vi "split_channels_syncBeforecnt.vi"(7 "last_sync_num_in":i32, 8 "error constant":errorcluster, 9 "sync_channel":u32, 10 "channels":u32[](array[numeric]), 11 "stamps":i64[](array[numeric])) -> (0 "error IO":errorcluster, 1 "time_delays":i64[](array[numeric]), 2 "n_sync":i32[](array[numeric]), 3 "count_channels":u32[](array[numeric]), 5 "last_sync_num_out":i32)   [LabVIEW 2018]
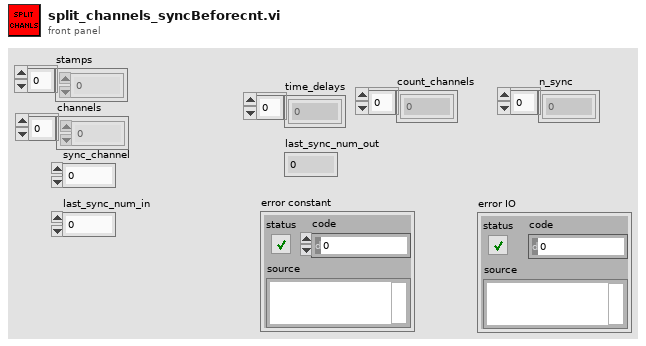
[diagram p1: front panel]
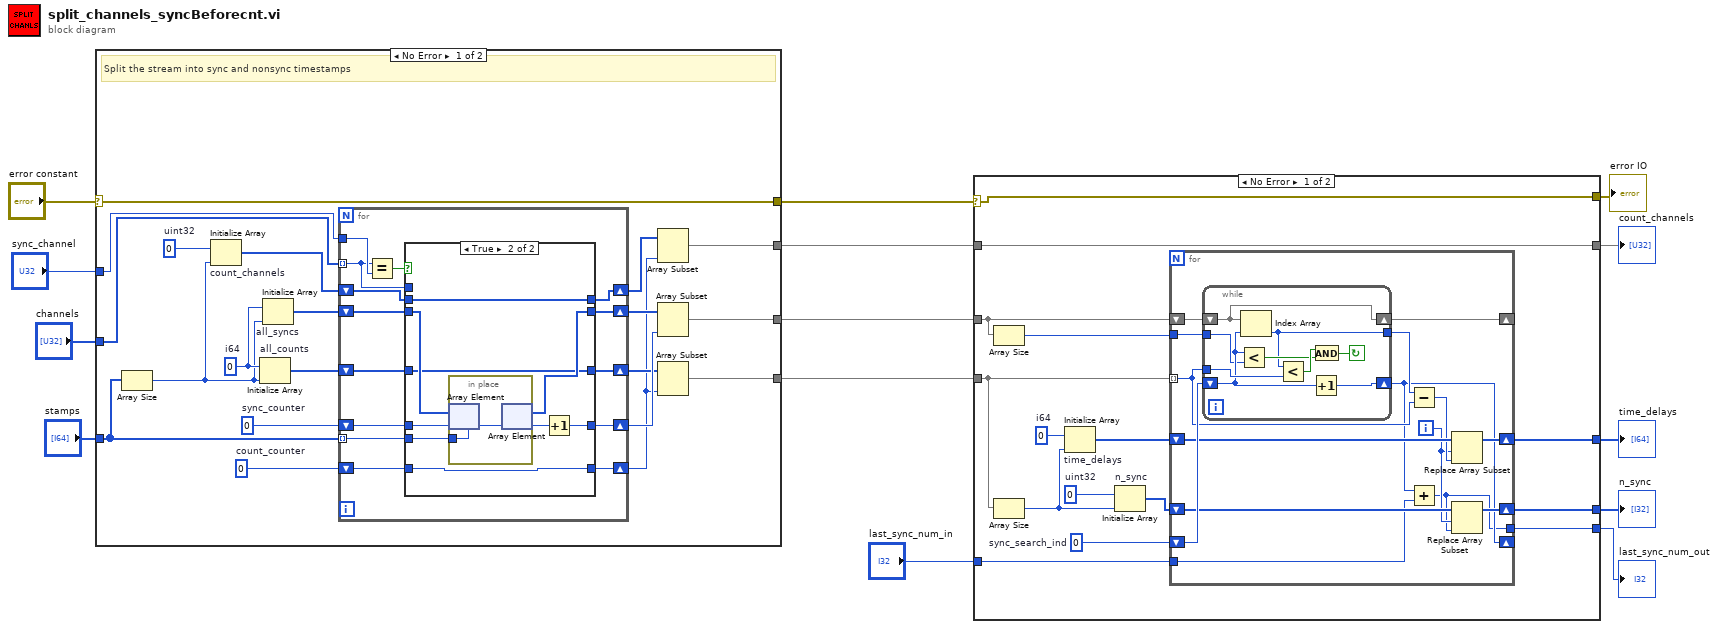
[diagram p0: block diagram]
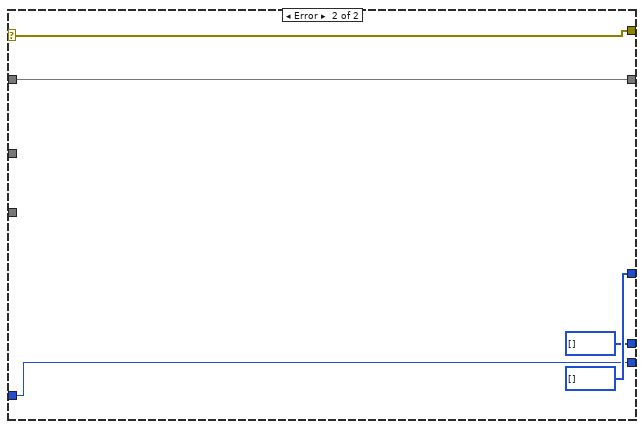
[diagram p2: hidden frame]
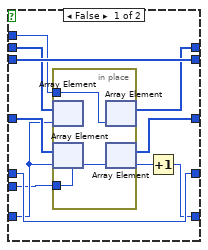
[diagram p3: hidden frame]
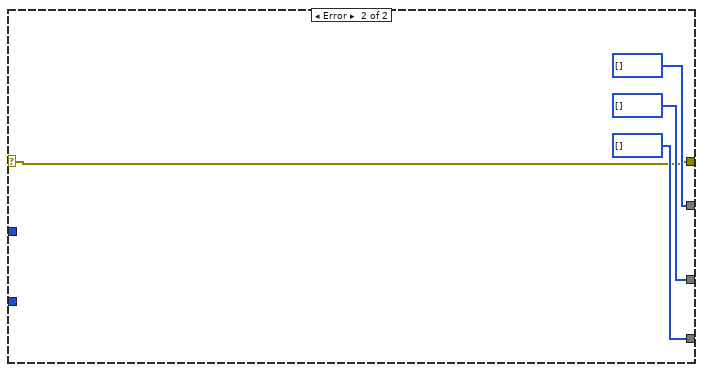
[diagram p4: hidden frame]
diagram:
  n1 = case shown="No Error" "error constant" {
    selector: "error constant" -> [w23 w72]
    tunnel: "channels" -> [w34 _]
    tunnel: "sync_channel" -> [w28 _]
    tunnel: "stamps" -> [w25 _]
    tunnel: [w23 w72] -> w10
    tunnel: [w20 i64[] []] -> w8
    tunnel: [w18 i64[] []] -> w9
    tunnel: [w15 u32[] []] -> w7
    frame No Error {
      w31 = 0  # count_counter
      w30 = 0  # sync_counter
      w26 = u32 0  # uint32
      w27 = i64 0  # i64
      # "Split the stream into sync and nonsync timestamps"
      n2 = Array Size(array=w25) -> (size(s)=w24:i32)
      n3 = Initialize Array "count_channels"(w26, w24) -> (w33:u32[])
      n4 = Initialize Array "all_counts"(w27, w24) -> (w32:i64[])
      n5 = Initialize Array "all_syncs"(w27, w24) -> (w29:i64[])
      n6 = for {
        tunnel: w25 -> [w35] mode=indexing
        tunnel: w28 -> [w48]
        shift-right: [w43] -> w22
        shift-left: w29 -> [w46]
        shift-right: [w44] -> w21
        shift-left: w30 -> [w45]
        shift-right: [w40] -> w16
        shift-left: w31 -> [w42]
        shift-right: [w39] -> w19
        shift-left: w32 -> [w41]
        shift-right: [w37] -> w17
        shift-left: w33 -> [w38]
        tunnel: w34 -> [w36] mode=indexing
        n7 = Equal?(x=w36, y=w48) -> (x = y?=w47:bool)
        n8 = case shown="True" w47 {
          tunnel: w46 -> [w59 w70]
          tunnel: w45 -> [w58 w69]
          tunnel: [w58 w67] -> w44
          tunnel: w36 -> [w49 _]
          tunnel: [w59 w66] -> w43
          tunnel: w42 -> [w52 w64]
          tunnel: w41 -> [w57 w65]
          tunnel: [w55 w64] -> w40
          tunnel: [w54 w65] -> w39
          tunnel: w38 -> [w53 w63]
          tunnel: [w51 w63] -> w37
          tunnel: w35 -> [w50 w62]
          frame False {
            n9 = in-place {
              in-place-border: w50 -> [w61]
              in-place-border: w49 -> [w60]
              n10 = in-place-array #1(w53, w52) -> ()  [unwired: 1 out]
              n11 = in-place-array #2(w57, w52) -> ()  [unwired: 1 out]
              n12 = in-place-array #1(w60) -> (w51:u32[])  [unwired: 1 out]
              n13 = in-place-array #2(w61) -> (w54:i64[], w56:i32)
            }
            n14 = Increment(x=w56) -> (x+1=w55:i32)
          }
          frame True {
            n15 = in-place {
              in-place-border: w62 -> [w71]
              n16 = in-place-array #3(w70, w69) -> ()  [unwired: 1 out]
              n17 = in-place-array #3(w71) -> (w66:i64[], w68:i32)
            }
            n18 = Increment(x=w68) -> (x+1=w67:i32)
          }
        }
      }
      n19 = Array Subset(array=w17, length=w16) -> (w15:u32[])  [unwired: 1 in]
      n20 = Array Subset(array=w22, length=w21) -> (w20:i64[])  [unwired: 1 in]
      n21 = Array Subset(array=w19, length=w16) -> (w18:i64[])  [unwired: 1 in]
    }
    frame Error {
    }
  }
  n22 = case shown="No Error" w10 {
    selector: w10 -> [w76 w115]
    tunnel: w9 -> [w86 _]
    tunnel: w8 -> [w83 _]
    tunnel: w7 -> [w90 w119]
    tunnel: [w90 w119] -> w6
    tunnel: [w81 i64[] []] -> w5
    tunnel: [w79 i32[] []] -> w4
    tunnel: "last_sync_num_in" -> [w78 w116]
    tunnel: [w77 w116] -> w2
    tunnel: [w76 w115] -> w1
    frame No Error {
      w85 = 0  # sync_search_ind
      w88 = 0  # uint32
      w89 = i64 0  # i64
      n23 = Array Size(array=w83) -> (size(s)=w82:i32)
      n24 = Array Size(array=w86) -> (size(s)=w87:i32)
      n25 = Initialize Array "time_delays"(w89, w87) -> (w84:i64[])
      n26 = Initialize Array "n_sync"(w88, w87) -> (w80:i32[])
      n27 = for {
        tunnel: w86 -> [w98] mode=indexing
        shift-right: [w102] -> _
        shift-left: w83 -> [w105]
        shift-right: [w100] -> w81
        shift-left: w84 -> [w101]
        shift-right: [w93] -> _
        shift-left: w85 -> [w104]
        tunnel: w82 -> [w103]
        shift-right: [w94] -> w79
        shift-left: w80 -> [w96]
        tunnel: w78 -> [w92]
        tunnel: [w91] -> w77
        i -> [w95]
        n28 = while {
          shift-right: [w107] -> w102
          shift-left: w105 -> [w107]
          shift-right: [w114] -> w93
          shift-left: w104 -> [w112]
          tunnel: w98 -> [w113]
          tunnel: w103 -> [w111]
          tunnel: [w106] -> w99
          stop <- w108 continue-if-true
          n29 = Less?(x=w112, y=w111) -> (x < y?=w109:bool)
          n30 = Index Array(array=w107, index=w112) -> (element=w106:i64)
          n31 = Less?(x=w106, y=w113) -> (x < y?=w110:bool)
          n32 = Increment(x=w112) -> (x+1=w114:i32)
          n33 = And(x=w110, y=w109) -> (x .and. y?=w108:bool)
        }
        n34 = Subtract(x=w99, y=w98) -> (x-y=w97:i64)
        n35 = Add(x=w93, y=w92) -> (x+y=w91:i32)
        n36 = Replace Array Subset(array=w101, new element=w97, index=w95) -> (w100:i64[])
        n37 = Replace Array Subset(array=w96, new element=w91, index=w95) -> (w94:i32[])
      }
    }
    frame Error {
    }
  }
  "count_channels" <- w6
  "time_delays" <- w5
  "n_sync" <- w4
  "last_sync_num_out" <- w2
  "error IO" <- w1
